vi "Buttons.vi"(4 "Button 8":bool, 5 "Button 1":bool, 6 "Button 7":bool, 7 "Button 2":bool, 8 "Button 6":bool, 9 "Button 5":bool, 10 "Button 4":bool, 11 "Button 3":bool) -> ()   [LabVIEW 2013]
uses:
  <vilib>/Rock Robotics/WPI/Solenoid/WPI_SolenoidValue.ctl
  <vilib>/Rock Robotics/WPI/Relay/WPI_RelayValue.ctl
  <vilib>/Rock Robotics/WPI/Solenoid/WPI_SolenoidSetEnum.vi
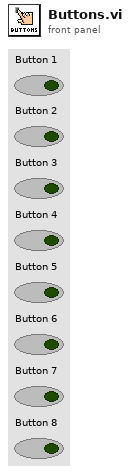
[diagram p1: front panel]
types:
  T1 = typedef "WPI_MotorControlDeviceRef.ctl" = cluster{"DeviceStatus":errorcluster, "Type":enum16{"PWM", "CAN"}, "PWM":cluster{"Digital Module":T2, "PWM Channel":T3, "DeadBand":T4}, "CAN":cluster{"Device Number":u8, "Control Mode":T5, "Semaphore":T6, "Max Vout":dbl}, "Invert":bool, "TransformRef":T7, "InvTransformRef":T7}
  T2 = typedef "FPGA_TypedefDigitalModule.ctl" = enum16{"Digital Module 1", "Digital Module 2"}
  T3 = typedef "FPGA_DIOPWMChannel.ctl" = enum8{"PWM 1", "PWM 2", "PWM 3", "PWM 4", "PWM 5", "PWM 6", "PWM 7", "PWM 8", "PWM 9", "PWM 10", "Invalid"}
  T4 = typedef "WPI_PWMDeadband.ctl" = cluster{"Name":string, "maxPositivePwm":i32, "minPositivePwm":i32, "centerPwm":i32, "maxNegativePwm":i32, "minNegativePwm":i32, "angularRange":u16}
  T5 = typedef "WPI_CANJaguar_ControlMode.ctl" = enum8{"Percent VBus", "Current", "Speed", "Position", "Voltage"}
  T6 = typedef "Semaphore RefNum" = refnum<k1>
  T7 = typedef "WPI_PWMTransform_ConPane.ctl" = refnum<vi>
  T8 = typedef "WPI_GyroDevRef.ctl" = cluster{"DevStatus":errorcluster, "Analog Module":T9, "Analog Channel":T10, "Offset":dbl, "Gain (VoltsPerDegree/Second)":dbl}
  T9 = typedef "FPGA_TypedefAnalogModule.ctl" = enum16{"Analog Module 1", "Analog Module 2"}
  T10 = typedef "FPGA_AIChannel.ctl" = enum8{"AI 1", "AI 2", "AI 3", "AI 4", "AI 5", "AI 6", "AI 7", "AI 8", "Invalid"}
  T11 = typedef "WPI_RelayValue.ctl" = enum16{"Off", "On", "Forward", "Reverse"}
  T12 = typedef "WPI_RelayDevRef.ctl" = cluster{"DevStatus":errorcluster, "Relay Channel":T13, "Digital Module":T2, "Relay Direction":T14}
  T13 = typedef "FPGA_DIORelayChannel.ctl" = enum8{"Relay 1", "Relay 2", "Relay 3", "Relay 4", "Relay 5", "Relay 6", "Relay 7", "Relay 8", "Invalid"}
  T14 = typedef "WPI_RelayDirection.ctl" = enum16{"Both directions", "Forward only", "Reverse only"}
  T15 = typedef "WPI_SolenoidValue.ctl" = enum16{"Off", "On", "Forward", "Reverse"}
  T16 = typedef "WPI_SolenoidDevRef.ctl" = cluster{"DevStatus":errorcluster, "Solenoid Module":T17, "Forward Solenoid Channel":T18, "Reverse Solenoid Channel":T18}
  T17 = typedef "FPGA_TypedefSolenoidModule.ctl" = enum16{"Solenoid Module 1", "Solenoid Module 2"}
  T18 = typedef "WPI_SolenoidChannel.ctl" = enum8{"Solenoid 1", "Solenoid 2", "Solenoid 3", "Solenoid 4", "Solenoid 5", "Solenoid 6", "Solenoid 7", "Solenoid 8", "Invalid"}
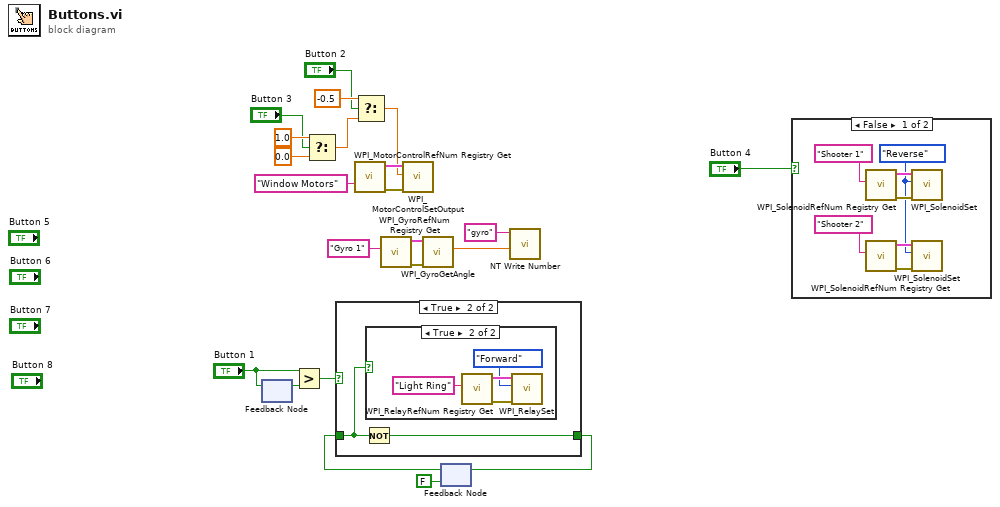
[diagram p0: block diagram]
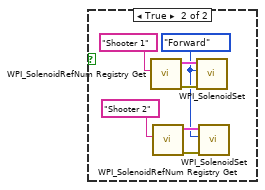
[diagram p2: hidden frame]
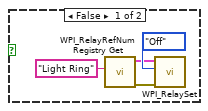
[diagram p4: hidden frame]
diagram:
  n1 = feedback #1() -> (w13:bool)  [unwired: 1 in]
  n2 = feedback-in #1("Button 1") -> ()
  n3 = Greater?(x="Button 1", y=w13) -> (0:w14:bool)
  n4 = Select(t=1.0, s="Button 3", f=0.0) -> (s? t:f=w16:dbl)
  n5 = call <vilib>:"WPI_MotorControlRefNum Registry Get.vi"("refnum name"="Window Motors") -> ("error out"=w22:errorcluster, "MotorControlDevRef"=w21:T1)  [unwired: 9 in]
  n6 = Select(t=-0.5, s="Button 2", f=w16) -> (s? t:f=w15:dbl)
  n7 = call <vilib>:"WPI_GyroRefNum Registry Get.vi"("refnum name"="Gyro 1") -> ("error out"=w9:errorcluster, "GyroDevRef"=w8:T8)  [unwired: 9 in]
  n8 = call <vilib>:"WPI_MotorControlSetOutput.vi"("error in (no error)"=w22, "Output"=w15, "MotorControlDevRef"=w21) -> ()  [unwired: 6 in, 3 out]
  n9 = call <vilib>:"WPI_GyroGetAngle.vi"("error in (no error)"=w9, "GyroDevRef"=w8) -> ("Angle"=w7:dbl)  [unwired: 6 in, 3 out]
  n10 = feedback #2(FALSE) -> (w11:bool)
  n11 = case shown="True" w14 {
    tunnel: [w23 w25] -> w12
    tunnel: w11 -> [w23 w24]
    frame False {
    }
    frame True {
      n12 = Not(x=w24) -> (.not. x?=w25:bool)
      n13 = case shown="True" w24 {
        frame False {
          n14 = call <vilib>:"WPI_RelayRefNum Registry Get.vi"("refnum name"="Light Ring") -> ("error out"=w26:errorcluster, "RelayDevRef"=w27:T12)  [unwired: 9 in]
          n15 = call <vilib>:"WPI_RelaySet.vi"("error in (no error)"=w26, "RelayValue"=WPI_RelayValue."Off", "RelayDevRef"=w27) -> ()  [unwired: 7 in, 2 out]
        }
        frame True {
          n16 = call <vilib>:"WPI_RelayRefNum Registry Get.vi"("refnum name"="Light Ring") -> ("error out"=w33:errorcluster, "RelayDevRef"=w32:T12)  [unwired: 9 in]
          n17 = call <vilib>:"WPI_RelaySet.vi"("error in (no error)"=w33, "RelayValue"=WPI_RelayValue."Forward", "RelayDevRef"=w32) -> ()  [unwired: 7 in, 2 out]
        }
      }
    }
  }
  n18 = feedback-in #2(w12) -> ()
  n19 = call <vilib>:"NT Write Number.vi"("Numeric"=w7, "Name"="gyro") -> ()  [unwired: 9 in, 1 out]
  n20 = case shown="False" "Button 4" {
    frame False {
      w34 = WPI_SolenoidValue."Reverse" ("Value")
      n21 = call <vilib>:"WPI_SolenoidRefNum Registry Get.vi"("refnum name"="Shooter 1") -> ("error out"=w40:errorcluster, "SolenoidDevRef"=w39:T16)  [unwired: 9 in]
      n22 = call <vilib>:"WPI_SolenoidRefNum Registry Get.vi"("refnum name"="Shooter 2") -> ("error out"=w37:errorcluster, "SolenoidDevRef"=w36:T16)  [unwired: 9 in]
      n23 = call-poly <vilib>:"WPI_SolenoidSet.vi"("error in (no error)"=w40, "Value"=w34, "SolenoidDevRef"=w39) -> ()  [unwired: 7 in, 2 out]
      n24 = call-poly <vilib>:"WPI_SolenoidSet.vi"("error in (no error)"=w37, "Value"=w34, "SolenoidDevRef"=w36) -> ()  [unwired: 7 in, 2 out]
    }
    frame True {
      w41 = WPI_SolenoidValue."Forward" ("Value")
      n25 = call <vilib>:"WPI_SolenoidRefNum Registry Get.vi"("refnum name"="Shooter 1") -> ("error out"=w47:errorcluster, "SolenoidDevRef"=w46:T16)  [unwired: 9 in]
      n26 = call <vilib>:"WPI_SolenoidRefNum Registry Get.vi"("refnum name"="Shooter 2") -> ("error out"=w44:errorcluster, "SolenoidDevRef"=w43:T16)  [unwired: 9 in]
      n27 = call-poly <vilib>:"WPI_SolenoidSet.vi"("error in (no error)"=w47, "Value"=w41, "SolenoidDevRef"=w46) -> ()  [unwired: 7 in, 2 out]
      n28 = call-poly <vilib>:"WPI_SolenoidSet.vi"("error in (no error)"=w44, "Value"=w41, "SolenoidDevRef"=w43) -> ()  [unwired: 7 in, 2 out]
    }
  }
